vi "Default Plugin Subpanel.vi"() -> ()   [LabVIEW 2021, in "CIF Manager UI.lvlib"]
uses:
  CIF Manager UI.lvlib
  CIFUI/Typedef/Class Data for SubPanel.ctl
  <vilib>/gRPC/LabVIEW gRPC Library/Shared/grpcId.ctl
  CIFUI/Typedef/Core UI References.ctl
  CIFUI/Typedef/Channel Connection.ctl
  CIFUI/Typedef/New Plugin.ctl
  CIFUI/Typedef/Run Listen Button.ctl
  CIFUI/Typedef/CIF_Manager_UI_Tab.ctl
  CIFUI/Typedef/SubPanel Events.ctl
  CIFUI/Typedef/New Connection Event Data.ctl
  CIFUI/Typedef/New Connection Plugin Event Data.ctl
  CIFUI/CIF_UI.lvclass
  CIFUI/CIF_UI.lvclass/CIF_UI.ctl
  CIFUI/Utilities/Get Human Readable Error.vi
  Plugins/Template/Grpc/Template_wrapper/TemplateWrapper.lvlib
  CIFCore/Grpc/CIFCoreWrapper/CIFCoreWrapper.lvlib
  <vilib>/gRPC/LabVIEW gRPC Library/grpc-lvsupport-release.lvlib
panel:
  in  "Update Config":bool
  in  "Class Data for SubPanel":T1
  in  "New Config":string
  out "Current Config":string
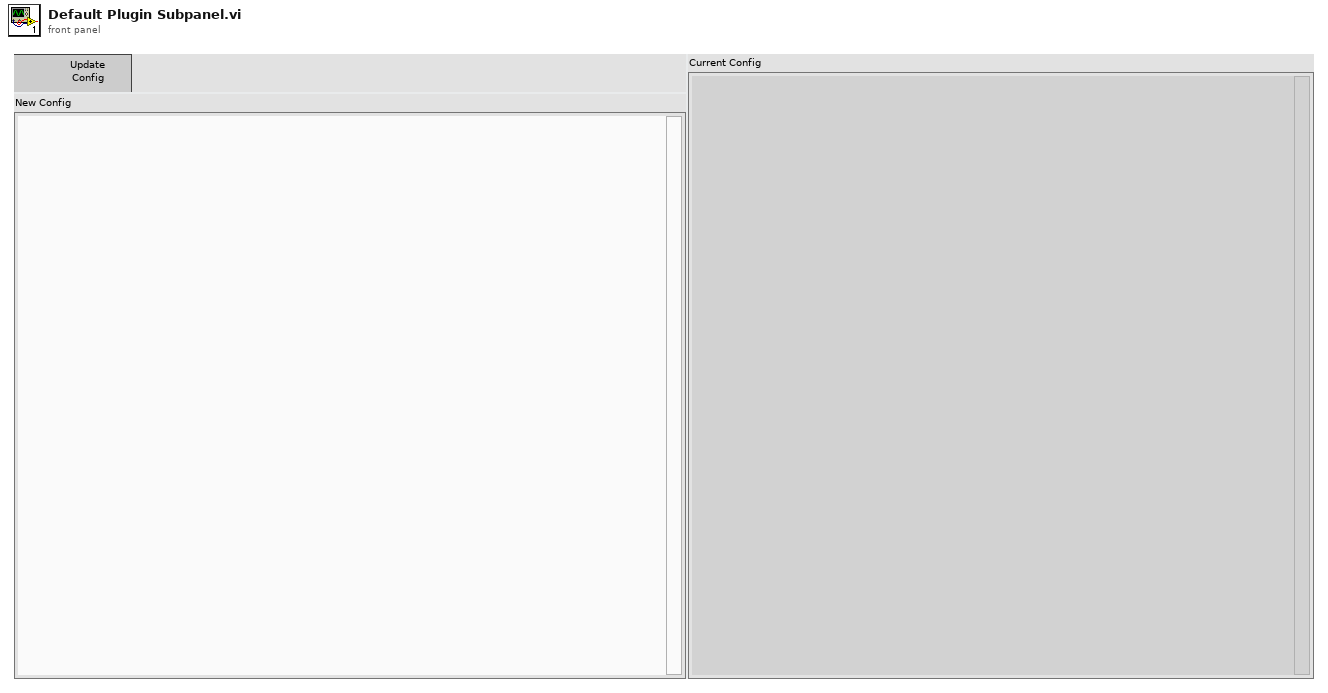
[diagram p1: front panel]
types:
  T1 = typedef "CIF_UI.lvclass/Class Data for SubPanel.ctl" = cluster{"IP Address":string, "Manager gRPC ID":T2, "Server Certificate File (.crt)":path, "Connected":bool, "Manager Connection":bool, "Core UI References":T3, "Subpanel Events":T4}
  T2 = typedef "grpc-lvsupport-release.lvlib/grpcId.ctl" = u64
  T3 = typedef "CIF_UI.lvclass/Core UI References.ctl" = cluster{"Discovered Plugins":refnum<vi>, "Discovered Plugins Valid":bool, "Loaded Plugins":refnum<vi>, "Loaded Plugins Valid":bool, "Publisher Channels":refnum<vi>, "Publisher Channels Valid":bool, "Subscriber Channels":refnum<vi>, "Subscriber Channels Valid":bool, "Plugin Status":refnum<vi>, "Plugin Status Valid":bool, "Channel Connection":refnum<vi>, "Channel Connection Valid":bool, "New Plugin Load":refnum<vi>, "New Plugin Load Valid":bool, "Errors":refnum<vi>, "Errors Valid":bool, "Plugin to Abort":refnum<vi>, "Plugin to Abort Valid":bool, "Connection":refnum<vi>, "Connection Valid":bool, "Exit":refnum<vi>, "Exit Valid":bool, "Run Listen":refnum<vi>, "Run Listen Valid":bool, "CIF Manager Tab":refnum<vi>, "Manger Tab Valid":bool, "Clear Local Error":refnum<vi>, "Clear Local Error Valid":bool, "Local Error":refnum<vi>, "Local Error Valid":bool, "System Errors":refnum<vi>, "System Errors Valid":bool, "Plugin Selection":refnum<vi>, "Plugin Selection Valid":bool}
  T4 = typedef "CIF_UI.lvclass/SubPanel Events.ctl" = cluster{"Clear Local Error":refnum<user-event>, "Shutdown":refnum<user-event>, "gRPC Connection":refnum<user-event>, "Plugin Connection":refnum<user-event>}
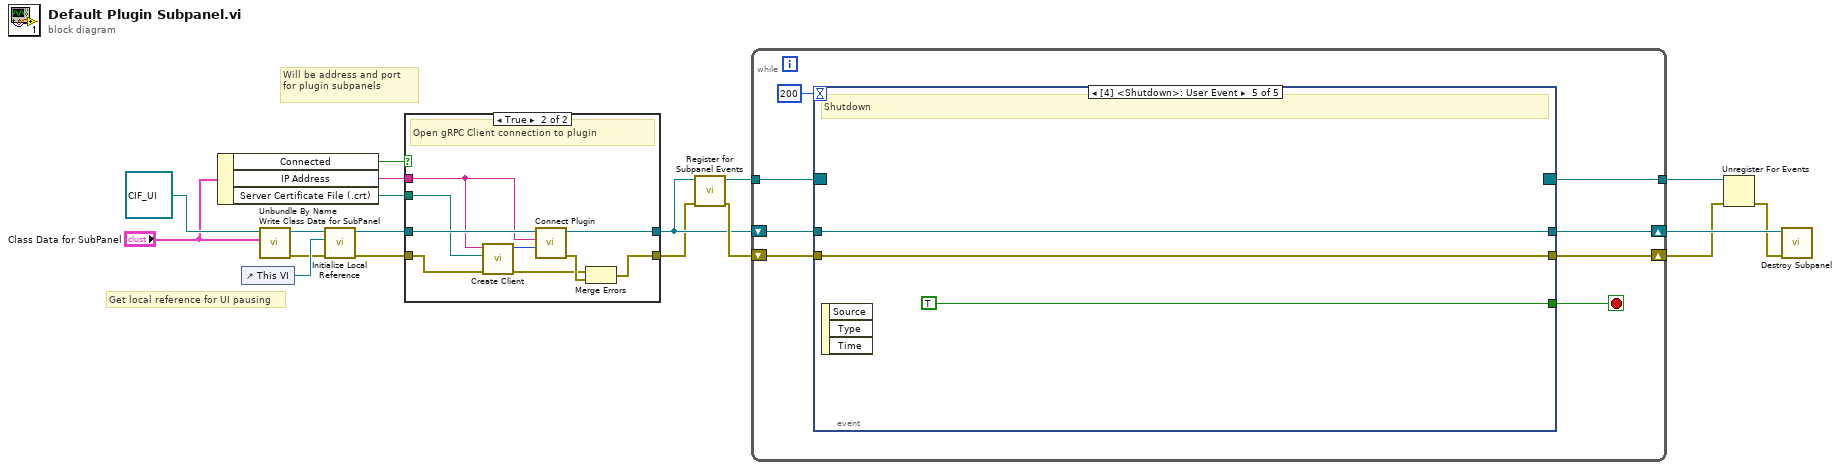
[diagram p0: block diagram]
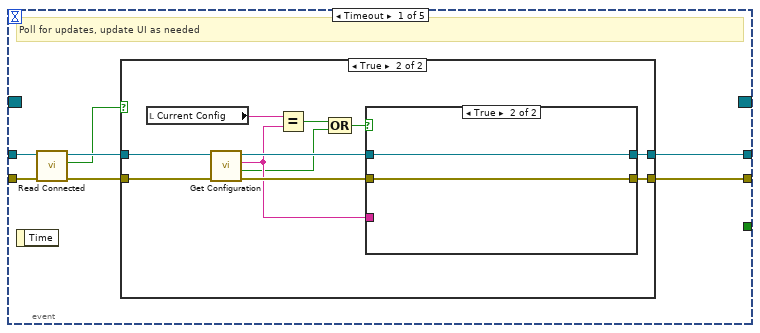
[diagram p3: hidden frame]
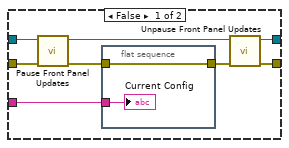
[diagram p5: hidden frame]
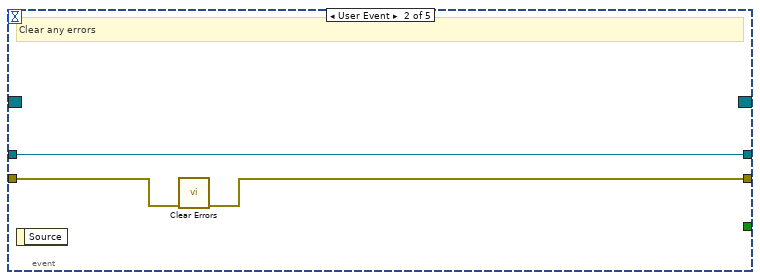
[diagram p6: hidden frame]
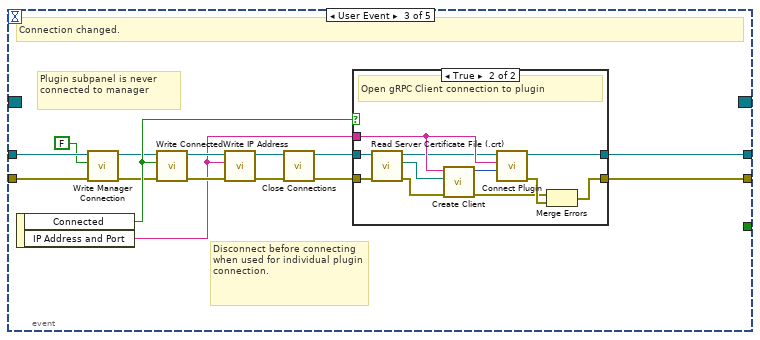
[diagram p7: hidden frame]
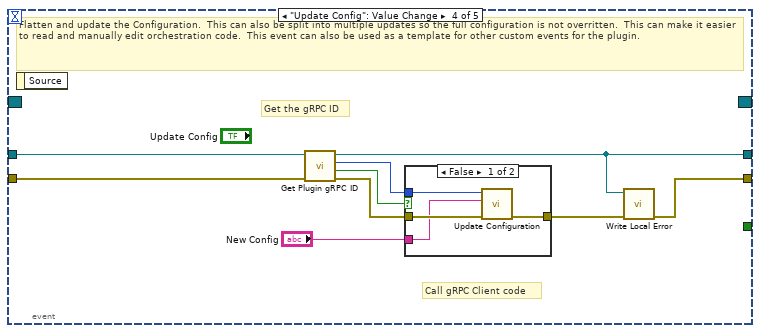
[diagram p9: hidden frame]
diagram:
  # "Will be address and port for plugin subpanels"
  # "Get local reference for UI pausing"
  n1 = Unbundle By Name("Class Data for SubPanel") -> ("Connected"=w3:bool, "IP Address"=w2:string, "Server Certificate File (.crt)"=w1:path)
  n2 = control-ref of="This VI"() -> (w18:refnum<vi>)
  n3 = call "Write Class Data for SubPanel.vi"("Class Data for SubPanel"="Class Data for SubPanel", "CIF_UI in"=refnum<class "CIF_UI.lvclass"> refnum) -> ("error out"=w9:errorcluster, "CIF_UI out"=w11:refnum<class "CIF_UI.lvclass">)  [unwired: 8 in]
  n4 = call "Initialize Local Reference.vi"("error in (no error)"=w9, "This VI"=w18, "CIF_UI in"=w11) -> ("error out"=w7:errorcluster, "CIF_UI out"=w8:refnum<class "CIF_UI.lvclass">)  [unwired: 7 in]
  n5 = case shown="True" w3 {
    tunnel: [w19 w29] -> w5
    tunnel: [w20 w27] -> w6
    tunnel: w8 -> [w20 w26]
    tunnel: w7 -> [w19 w25]
    tunnel: w2 -> [_ w22]
    tunnel: w1 -> [_ w21]
    frame False {
    }
    frame True {
      # "Open gRPC Client connection to plugin"
      n6 = call "Create Client.vi"("error in"=w25, "Server Certificate File (.crt)"=w21, "address"=w22) -> ("error out"=w24:errorcluster, "gRPC ID Out"=w23:T2)  [unwired: 7 in]
      n7 = call "Connect Plugin.vi"("gRPC ID"=w23, "Address"=w22, "CIF_UI in"=w26) -> ("error out"=w28:errorcluster, "CIF_UI out"=w27:refnum<class "CIF_UI.lvclass">)  [unwired: 7 in]
      n8 = Merge Errors(w24, w28) -> (w29:errorcluster)
    }
  }
  n9 = call "Register for Subpanel Events.vi"("error in (no error)"=w5, "CIF_UI in"=w6) -> ("error out"=w16:errorcluster, "Event Registration Refnum"=w17:refnum<event-registration>)  [unwired: 8 in]
  n10 = while {
    tunnel: w17 -> [w36]
    shift-right: [w31] -> w15
    shift-left: w6 -> [w34]
    shift-right: [w32] -> w13
    shift-left: w16 -> [w33]
    tunnel: [w30] -> w14
    stop <- w35 stop-if-true
    n11 = event shown="[4] <Shutdown>: User Event" {
      selector: w36 -> [_ _ _ _ _]
      dyn-events: [_ _ _ _ _] -> w30
      timeout: 200 -> [_ _ _ _ _]
      tunnel: [_ _ _ _ TRUE] -> w35
      tunnel: w34 -> [w40 w70 w77 w105 w116]
      tunnel: w33 -> [w41 w72 w76 w101 w115]
      tunnel: [w38 w71 w78 w109 w115] -> w32
      tunnel: [w39 w70 w79 w104 w116] -> w31
      event Timeout {
        # "Poll for updates, update UI as needed"
        n12 = event-data() -> ()  [unwired: 1 in, 1 out]
        n13 = call "Read Connected.vi"("error in (no error)"=w41, "CIF_UI in"=w40) -> ("error out"=w43:errorcluster, "Connected"=w42:bool, "CIF_UI out"=w44:refnum<class "CIF_UI.lvclass">)  [unwired: 7 in]
        n14 = case shown="True" w42 {
          tunnel: w43 -> [w45 w54]
          tunnel: [w45 w57] -> w38
          tunnel: w44 -> [w46 w55]
          tunnel: [w46 w56] -> w39
          frame False {
          }
          frame True {
            n15 = local read "Current Config"() -> (w51:string)
            n16 = call "Get Configuration.vi"("error in (no error)"=w54, "CIF_Plugin_UI in"=w55) -> ("error out"=w52:errorcluster, "Not Found"=w48:bool, "JSON Configuration"=w50:string, "CIF_Plugin_UI out"=w53:refnum<class "CIF_UI.lvclass">)  [unwired: 6 in]
            n17 = Equal?(x=w51, y=w50) -> (x = y?=w49:bool)
            n18 = Compound Arithmetic op=OR(w49, w48) -> (w47:bool)
            n19 = case shown="True" w47 {
              tunnel: [w65 w68] -> w57
              tunnel: [w64 w69] -> w56
              tunnel: w53 -> [w63 w69]
              tunnel: w52 -> [w62 w68]
              tunnel: w50 -> [w58 _]
              frame False {
                n20 = call "Pause Front Panel Updates.vi"("error in (no error)"=w62, "CIF_UI in"=w63) -> ("error out"=w60:errorcluster, "CIF_UI out"=w61:refnum<class "CIF_UI.lvclass">)  [unwired: 8 in]
                n21 = flat-sequence {
                  tunnel: w60 -> [w67]
                  tunnel: [w67] -> w59
                  tunnel: w58 -> [w66]
                  frame #0 {
                    "Current Config" <- w66
                  }
                }
                n22 = call "Unpause Front Panel Updates.vi"("error in (no error)"=w59, "CIF_UI in"=w61) -> ("error out"=w65:errorcluster, "CIF_UI out"=w64:refnum<class "CIF_UI.lvclass">)  [unwired: 8 in]
              }
              frame True {
              }
            }
          }
        }
      }
      event User Event {
        # "Clear any errors"
        n23 = event-data() -> ()  [unwired: 1 in, 1 out]
        n24 = call <vilib>:"Clear Errors.vi"("error in (no error)"=w72) -> ("error out"=w71:errorcluster)  [unwired: 5 in, 1 out]
      }
      event User Event {
        # "Plugin subpanel is never connected to manager"
        # "Disconnect before connecting when used for individual plugin connection."
        # "Connection changed."
        n25 = event-data() -> ("Connected"=w80:bool, "IP Address and Port"=w81:string)  [unwired: 1 in]
        n26 = call "Write Manager Connection.vi"("error in (no error)"=w76, "Manager Connection"=FALSE, "CIF_UI in"=w77) -> ("error out"=w74:errorcluster, "CIF_UI out"=w75:refnum<class "CIF_UI.lvclass">)  [unwired: 7 in]
        n27 = call "Write Connected.vi"("error in (no error)"=w74, "Connected"=w80, "CIF_UI in"=w75) -> ("error out"=w86:errorcluster, "CIF_UI out"=w87:refnum<class "CIF_UI.lvclass">)  [unwired: 7 in]
        n28 = call "Write IP Address.vi"("error in (no error)"=w86, "IP Address"=w81, "CIF_UI in"=w87) -> ("error out"=w84:errorcluster, "CIF_UI out"=w85:refnum<class "CIF_UI.lvclass">)  [unwired: 7 in]
        n29 = call "Close Connections.vi"("error in (no error)"=w84, "CIF_UI in"=w85) -> ("error out"=w82:errorcluster, "CIF_UI out"=w83:refnum<class "CIF_UI.lvclass">)  [unwired: 8 in]
        n30 = case shown="True" w80 {
          tunnel: [w88 w100] -> w78
          tunnel: [w89 w98] -> w79
          tunnel: w83 -> [w89 w94]
          tunnel: w82 -> [w88 w93]
          tunnel: w81 -> [_ w95]
          frame False {
          }
          frame True {
            # "Open gRPC Client connection to plugin"
            n31 = call "Read Server Certificate File (.crt).vi"("error in (no error)"=w93, "CIF_UI in"=w94) -> ("error out"=w91:errorcluster, "Server Certificate File (.crt)"=w90:path, "CIF_UI out"=w92:refnum<class "CIF_UI.lvclass">)  [unwired: 7 in]
            n32 = call "Create Client.vi"("error in"=w91, "Server Certificate File (.crt)"=w90, "address"=w95) -> ("error out"=w97:errorcluster, "gRPC ID Out"=w96:T2)  [unwired: 7 in]
            n33 = call "Connect Plugin.vi"("gRPC ID"=w96, "Address"=w95, "CIF_UI in"=w92) -> ("error out"=w99:errorcluster, "CIF_UI out"=w98:refnum<class "CIF_UI.lvclass">)  [unwired: 7 in]
            n34 = Merge Errors(w97, w99) -> (w100:errorcluster)
          }
        }
      }
      event "Update Config": Value Change {
        # "Call gRPC Client code"
        # "Get the gRPC ID"
        # "Flatten and update the Configuration.  This can also be split into multiple updates so the full configuration is not overritten.  This can make it easier to read and manually edit orchestration code.  This event can also be used as a template for other custom events for the plugin."
        n35 = event-data() -> ()  [unwired: 1 in, 1 out]
        n36 = call "Get Plugin gRPC ID.vi"("error in (no error)"=w101, "CIF_UI in"=w105) -> ("error out"=w106:errorcluster, "Not Found"=w107:bool, "gRPC ID"=w108:T2, "CIF_UI out"=w104:refnum<class "CIF_UI.lvclass">)  [unwired: 5 in, 1 out]
        n37 = case shown="False" w107 {
          tunnel: w108 -> [w113 _]
          tunnel: w106 -> [w112 w114]
          tunnel: [w111 w114] -> w103
          tunnel: "New Config" -> [w110 _]
          frame False {
            n38 = call "Update Configuration.vi"("error in"=w112, "JSON Configuration"=w110, "gRPC ID"=w113) -> ("error out"=w111:errorcluster)  [unwired: 7 in, 1 out]
          }
          frame True {
          }
        }
        n39 = call "Write Local Error.vi"("error in (no error)"=w103, "CIF_UI in"=w104) -> ("error out"=w109:errorcluster)  [unwired: 9 in]
      }
      event User Event {
        # "Shutdown"
        n40 = event-data() -> ()  [unwired: 1 in, 3 out]
      }
    }
  }
  n41 = Unregister For Events(event registration refnum=w14, error in=w13) -> (error out=w12:errorcluster)
  n42 = call "Destroy Subpanel.vi"("error in (no error)"=w12, "CIF_UI in"=w15) -> ()  [unwired: 8 in, 2 out]
